vi "Last Updated Sort.vi"(11 "list in":T1[](array[typedef]) {"Creation Date" format="%<%x>T"; "Last Updated" format="%<%x>T"}) -> (3 "Array":T1[](array[typedef]) {"Creation Date" format="%<%x>T"; "Last Updated" format="%<%x>T"})   [LabVIEW 2018]
uses:
  Type Defs/SR Cluster.ctl
  Type Defs/SR Status.ctl
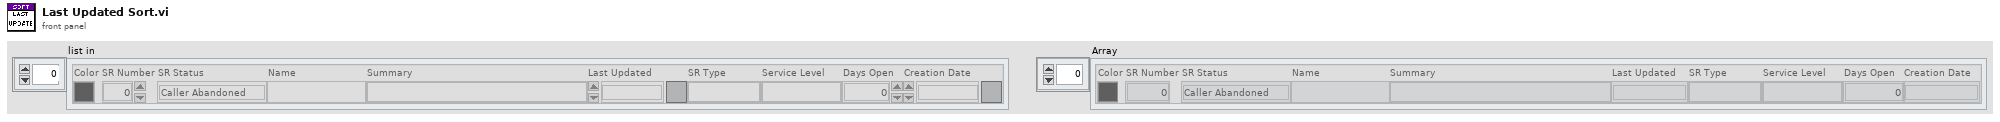
[diagram p1: front panel]
types:
  T1 = typedef "SR Cluster.ctl" = cluster{"Color":u32, "SR Number":i32, "SR Status":T2, "Name":string, "Summary":string, "Last Updated":timestamp, "SR Type":string, "Service Level":string, "Days Open":dbl, "Creation Date":timestamp}
  T2 = typedef "SR Status.ctl" = enum16{"Caller Abandoned", "Created in Error", "Expired", "Forum Resolved AE", "Forum Resolved Customer", "IN WORK", "IN WORK Collab with AES", "IN WORK Collab with PSE", "IN WORK Collab with SE", "IN WORK Customer Added Note", "IN WORK Escalation", "IN WORK Wait on Customer", "Open", "Potentially Resolved", "Presumed Resolved", "RMA Approved for Return", "RMA Closed", "RMA Closed - DOA", "RMA In Progress", "RMA Open", "RMA Waiting on Customer", "Resolved", "Passed Off"}
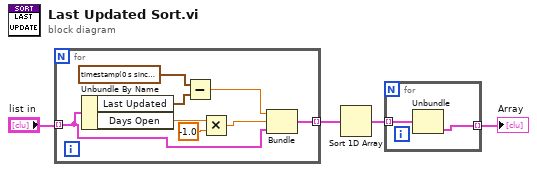
[diagram p0: block diagram]
diagram:
  n1 = for {
    tunnel: "list in" -> [w5] mode=indexing
    tunnel: [w12] -> w1 mode=indexing
    n2 = Unbundle By Name(w5) -> ("Last Updated"=w11:timestamp, "Days Open"=w8:dbl)
    n3 = Subtract(x=timestamp(0 s since 1904-01-01) ("Last Updated"), y=w11) -> (x-y=w9:dbl)
    n4 = Multiply(x=w8, y=-1.0) -> (x*y=w7:dbl)
    n5 = Bundle(w9, w7, "SR Cluster"=w5) -> (w12:cluster{dbl, dbl, "SR Cluster":T1})  [unwired: 1 in]
  }
  n6 = Sort 1D Array(array=w1) -> (sorted array=w2:cluster{dbl, dbl, "SR Cluster":T1}[])
  n7 = for {
    tunnel: w2 -> [w14] mode=indexing
    tunnel: [w13] -> w4 mode=indexing
    n8 = Unbundle(w14) -> ("SR Cluster"=w13:T1)  [unwired: 2 out]
  }
  "Array" <- w4
